vi "PatternMatch_ReadTemplate.vi"(8 "error in (no error)":errorcluster, 10 "template path":path, 11 "Template":T1) -> (0 "error out":errorcluster, 3 "Template Out":T1)   [LabVIEW 2019]
uses:
  <vilib>/vision/Image Controls.llb/IMAQ Image.ctl
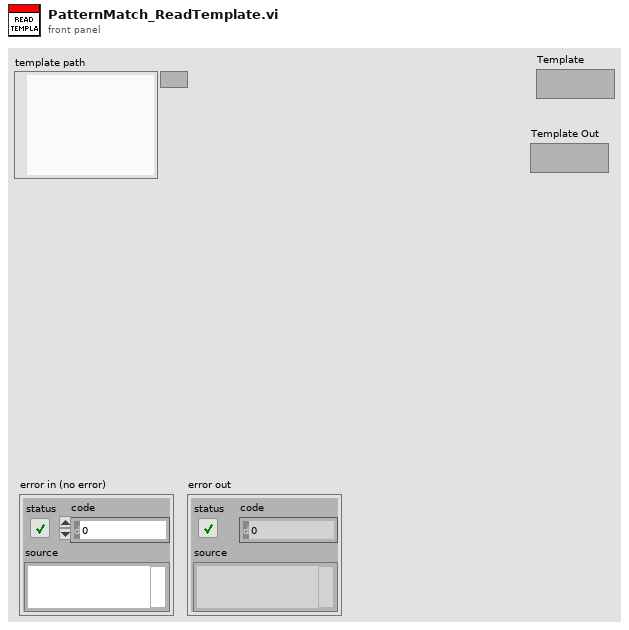
[diagram p1: front panel]
types:
  T1 = typedef "IMAQ Image.ctl" = refnum<image>
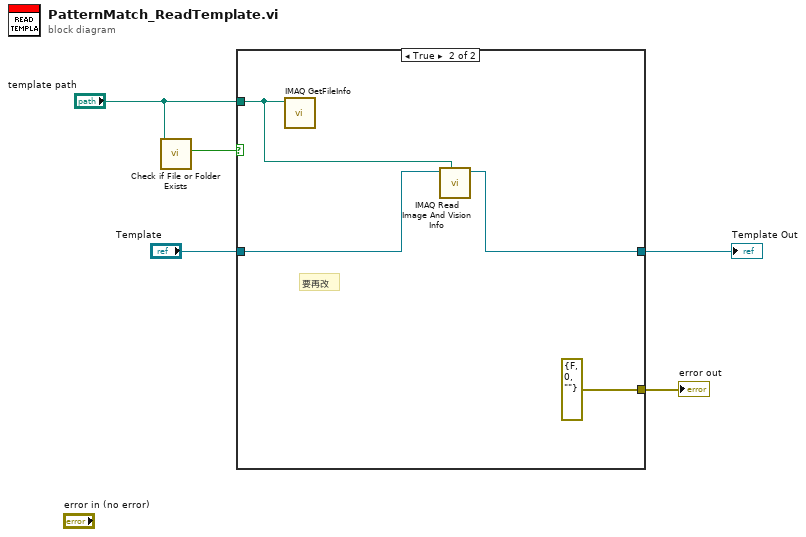
[diagram p0: block diagram]
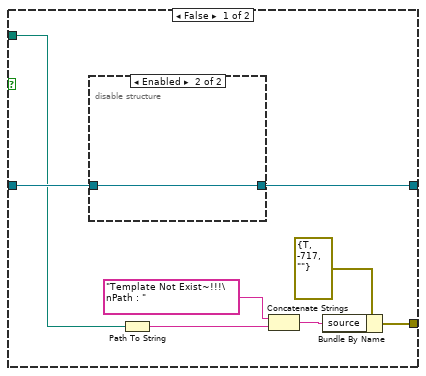
[diagram p2: hidden frame]
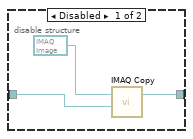
[diagram p3: hidden frame]
diagram:
  n1 = call <vilib>:"Check if File or Folder Exists.vi"("path"="template path") -> ("file or folder exists?"=w5:bool)  [unwired: 8 in, 2 out]
  n2 = case shown="True" w5 {
    tunnel: "Template" -> [w13 w21]
    tunnel: [w12 w19] -> w3
    tunnel: "template path" -> [w7 w20]
    tunnel: [w10 errorcluster {"status"=FALSE, "code"=0, "source"=""} ("error out")] -> w1
    frame False {
      n3 = disable-structure shown="Enabled" {
        disable-tunnel: w13 -> [w15 w17]
        disable-tunnel: [w14 w17] -> w12
        frame Disabled {
          n4 = call "IMAQ Copy"("Image Dst"=w15, "Image Src"=T1 refnum) -> ("Image Dst Out"=w14:T1)  [unwired: 4 in, 1 out]
        }
        frame Enabled {
        }
      }
      n5 = Path To String(path=w7) -> (string=w6:string)
      n6 = Concatenate Strings("Template Not Exist~!!!\nPath : " ("source"), w6) -> (w8:string)
      n7 = Bundle By Name(cluster=errorcluster {"status"=TRUE, "code"=-717, "source"=""} ("error out"), "source"=w8) -> (w10:errorcluster)
    }
    frame True {
      # "要再改"
      n8 = call "IMAQ GetFileInfo"("File Path"=w20) -> ()  [unwired: 4 in, 7 out]
      n9 = call "IMAQ Read Image And Vision Info"("File Path"=w20, "Image"=w21) -> ("Image Out"=w19:T1)  [unwired: 7 in, 2 out]
    }
  }
  "error out" <- w1
  "Template Out" <- w3
